vi "adjust_manip_coordSystem.vi"(7 "which manipulator":T2(ring), 8 "error in":errorcluster, 9 "transform cluster + actuator":T1, 11 "pipette position difference (px)":dbl[](array[numeric])) -> (0 "error out":errorcluster)   [LabVIEW 2015]
uses:
  pipette cleaning/pressure box/cleaning_soft/controls/actuator_type.ctl
  pipette cleaning/pressure box/cleaning_soft/controls/actuator_cluster.ctl
  transform_properties_actuators.ctl
  controls/transform_cluster_actuator.ctl
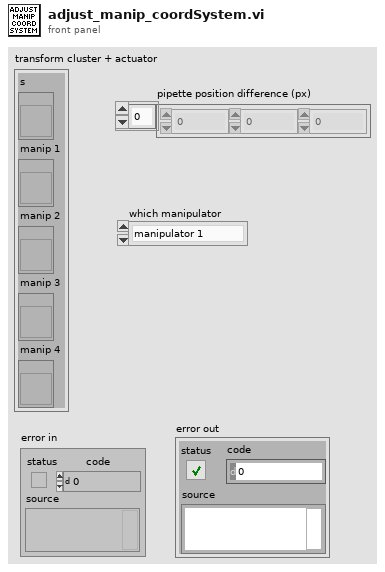
[diagram p1: front panel]
types:
  T1 = typedef "transform_cluster_actuator.ctl" = cluster{"s":refnum<vi>, "manip 1":refnum<vi>, "manip 2":refnum<vi>, "manip 3":refnum<vi>, "manip 4":refnum<vi>}
  T2 = enum16{"manipulator 1", "manipulator 2", "manipulator 3", "manipulator 4"}
  T3 = typedef "transform_properties_actuators.ctl" = cluster{"theta (deg)":dbl, "X sc factor (px/step)":dbl, "Y sc factor (px/step)":dbl, "zero loc (x,y,z)":dbl[], "flip y?":bool, "flip x?":bool, "gamma (deg)":dbl, "flip z?":bool, "Z sc factor (px/step)":dbl, "actuator":T4, "safe space (steps)":i32[]}
  T4 = typedef "actuator_cluster.ctl" = cluster{"Actuator COM":refnum<visa-resource-name>, "Actuator type":T5}
  T5 = typedef "actuator_type.ctl" = enum16{"Scientifica", "Sutter", "Demo", "Off"}
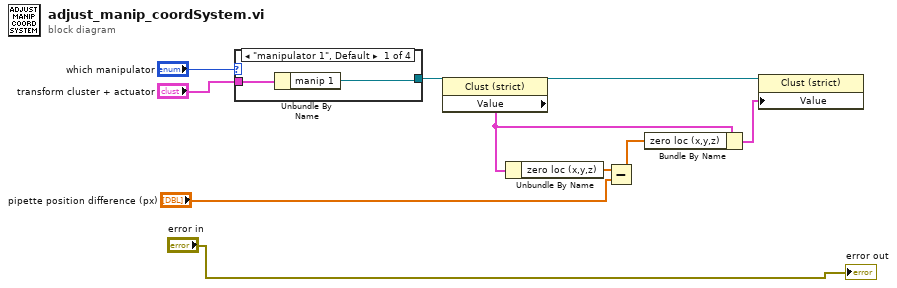
[diagram p0: block diagram]
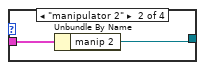
[diagram p2: hidden frame]
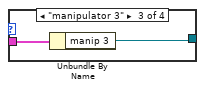
[diagram p3: hidden frame]
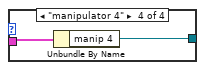
[diagram p4: hidden frame]
diagram:
  n1 = case shown="\"manipulator 1\", Default" "which manipulator" {
    tunnel: "transform cluster + actuator" -> [w12 w14 w16 w18]
    tunnel: [w11 w13 w15 w17] -> w9
    frame "manipulator 1", Default {
      n2 = Unbundle By Name(w12) -> ("manip 1"=w11:refnum<vi>)
    }
    frame "manipulator 2" {
      n3 = Unbundle By Name(w14) -> ("manip 2"=w13:refnum<vi>)
    }
    frame "manipulator 3" {
      n4 = Unbundle By Name(w16) -> ("manip 3"=w15:refnum<vi>)
    }
    frame "manipulator 4" {
      n5 = Unbundle By Name(w18) -> ("manip 4"=w17:refnum<vi>)
    }
  }
  n6 = property class="Clust (strict)"(reference=w9) -> (reference out=w7:refnum<vi>, "Value"=w6:T3)  [unwired: 1 in, 1 out]
  n7 = Unbundle By Name(w6) -> ("zero loc (x,y,z)"=w3:dbl[])
  n8 = Subtract(x=w3, y="pipette position difference (px)") -> (x-y=w4:dbl[])
  n9 = Bundle By Name(cluster=w6, "zero loc (x,y,z)"=w4) -> (w5:T3)
  n10 = property class="Clust (strict)"(reference=w7, "Value"=w5) -> ()  [unwired: 1 in, 2 out]
  "error out" <- "error in"
